vi "SignalGeneratorJ&J.vi"(9 "Amplitude":dbl, 10 "Frequency":dbl) -> ()   [LabVIEW 2015]
panel:
  in  "error in 2":errorcluster caption="error in"
  out "error out":errorcluster
  in  "Stop":bool
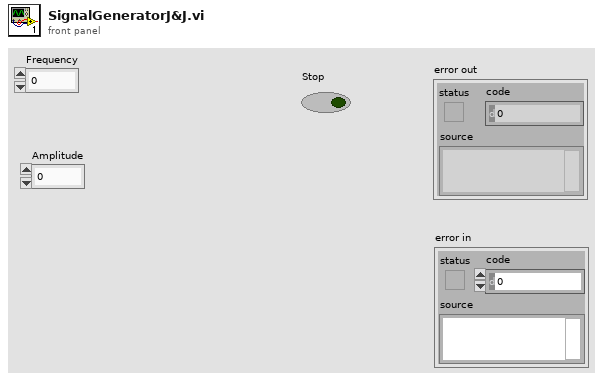
[diagram p1: front panel]
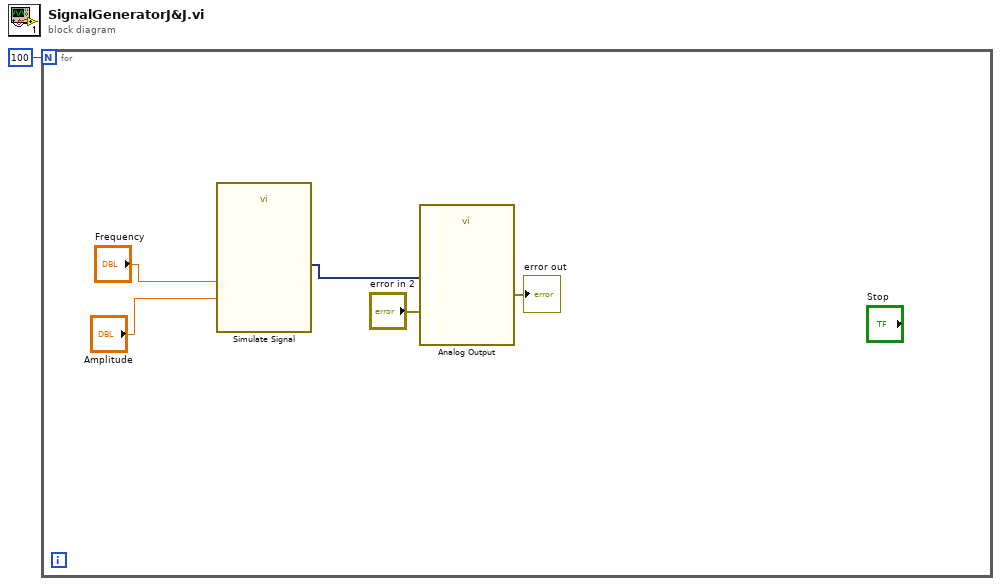
[diagram p0: block diagram]
diagram:
  n1 = for {
    N: 100 -> [_]
    n2 = call "Simulate Signal"("Frequency"="Frequency", "Amplitude"="Amplitude") -> ("Sine"=w6:dynamicdata)  [unwired: 12 in, 1 out]
    n3 = call "Analog Output"("data"=w6, "error in"="error in 2") -> ("error out"=→"error out":errorcluster)  [unwired: 15 in, 2 out]
  }
